vi "Create Rename if exists.vi"(8 "error in":errorcluster, 10 "Rename Name":string, 11 "Source Path":path) -> (0 "error out":errorcluster, 2 "created file":refnum<file>, 3 "created path":path)   [LabVIEW 2010]
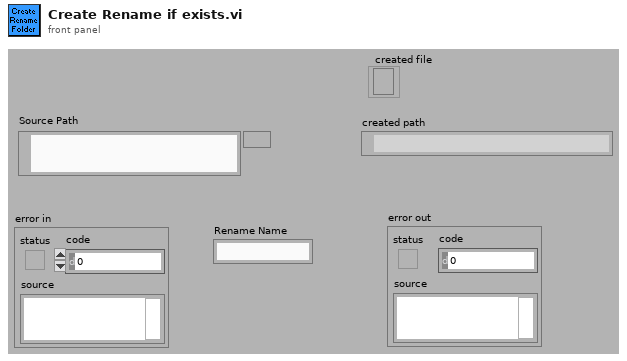
[diagram p1: front panel]
types:
  T1 = enum16{"open", "replace", "create", "open or create", "replace or create", "replace or create with confirmation"}
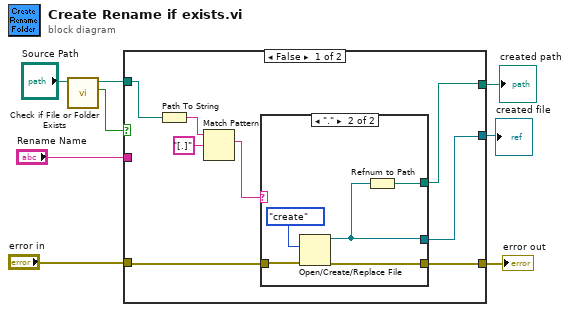
[diagram p0: block diagram]
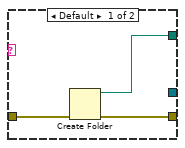
[diagram p2: hidden frame]
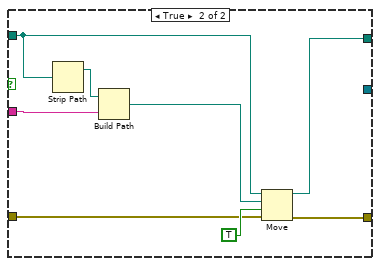
[diagram p3: hidden frame]
diagram:
  n1 = call <vilib>:"Check if File or Folder Exists.vi"("path"="Source Path") -> ("file or folder exists?"=w8:bool, "dup path"=w2:path)  [unwired: 8 in, 1 out]
  n2 = case shown="False" w8 {
    tunnel: w2 -> [w10 w32]
    tunnel: "error in" -> [w16 w26]
    tunnel: [w15 w25] -> w5
    tunnel: [w9 w27] -> w4
    tunnel: "Rename Name" -> [_ w29]
    tunnel: [w11 _] -> w1
    frame False {
      n3 = Path To String(path=w10) -> (string=w14:string)
      n4 = Match Pattern(string=w14, regular expression="[.]") -> (match substring=w12:string)  [unwired: 1 in, 3 out]
      n5 = case shown="\".\"" w12 {
        tunnel: w16 -> [w19 w23]
        tunnel: [w18 w22] -> w15
        tunnel: [_ w21] -> w11
        tunnel: [w17 w20] -> w9
        frame Default {
          n6 = Create Folder(error in=w19) -> (created path=w17:path, error out=w18:errorcluster)  [unwired: 2 in, 1 out]
        }
        frame "." {
          n7 = Open/Create/Replace File(error in=w23, operation (0:open)=T1."create") -> (refnum out=w21:refnum<file>, error out=w22:errorcluster)  [unwired: 4 in, 1 out]
          n8 = Refnum to Path(1:w21) -> (0:w20:path)
        }
      }
    }
    frame True {
      n9 = Strip Path(path=w32) -> (stripped path=w30:path)  [unwired: 1 out]
      n10 = Build Path(base path=w30, name or relative path=w29) -> (appended path=w28:path)
      n11 = Move(source path=w32, error in=w26, 9:TRUE ("overwrite (F)"), 10:w28) -> (error out=w25:errorcluster, 3:w27:path)  [unwired: 1 in, 1 out]
    }
  }
  "error out" <- w5
  "created path" <- w4
  "created file" <- w1
